vi "WinSSIZE_T.vi"() -> ()   [LabVIEW 2023]
doc: "This function squares the value of input and returns the value in output.\n\nFor information on the data types used for the DLL function, right-click on the Call Library Function node and choose Configure."
uses:
  CLF_Example.dll
panel:
  out "output":i64
  in  "input":i64=10
  # "See the block diagram for more information."
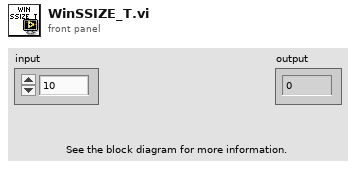
[diagram p1: front panel]
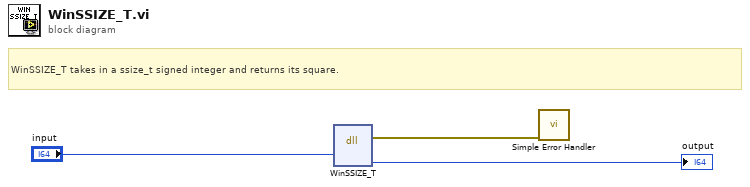
[diagram p0: block diagram]
diagram:
  # "WinSSIZE_T takes in a ssize_t signed integer and returns its square."
  n1 = dll-call lib="c:/dev/_r/4/eng/lv-core/lvpostprocessingd/lv_mc_x86_64/dist_i386/examples/Connectivity/Libraries and Executables/DLL Calling VIs/CLF_Example**.*" fn="WinSSIZE_T"("input"="input") -> (error out=w1:errorcluster, "output"=→"output":i64)  [unwired: 3 in, 4 out]
  n2 = call <vilib>:"Simple Error Handler.vi"("error in (no error)"=w1) -> ()  [unwired: 4 in, 5 out]
